vi "Thread@SubThreadSuspend__Parameter.vi"(1 "ParamterIn":string) -> (0 "ParamterOut":string)   [LabVIEW 2020]
panel:
  out "SubThread Name":string[](array[string])
  in  "ALL":bool
  in  "Thread Label":string(combo)
  in  "Confirm":bool
  # "Thread@SubThreadSuspend $SubName1(,$SubName2....)\nThread@SubThreadSuspend ALL\nThread@SubThreadSuspend ALL(,$SubName1,$SubName2....)"
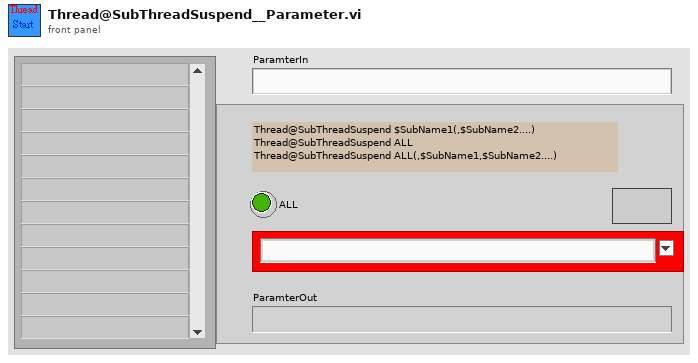
[diagram p1: front panel]
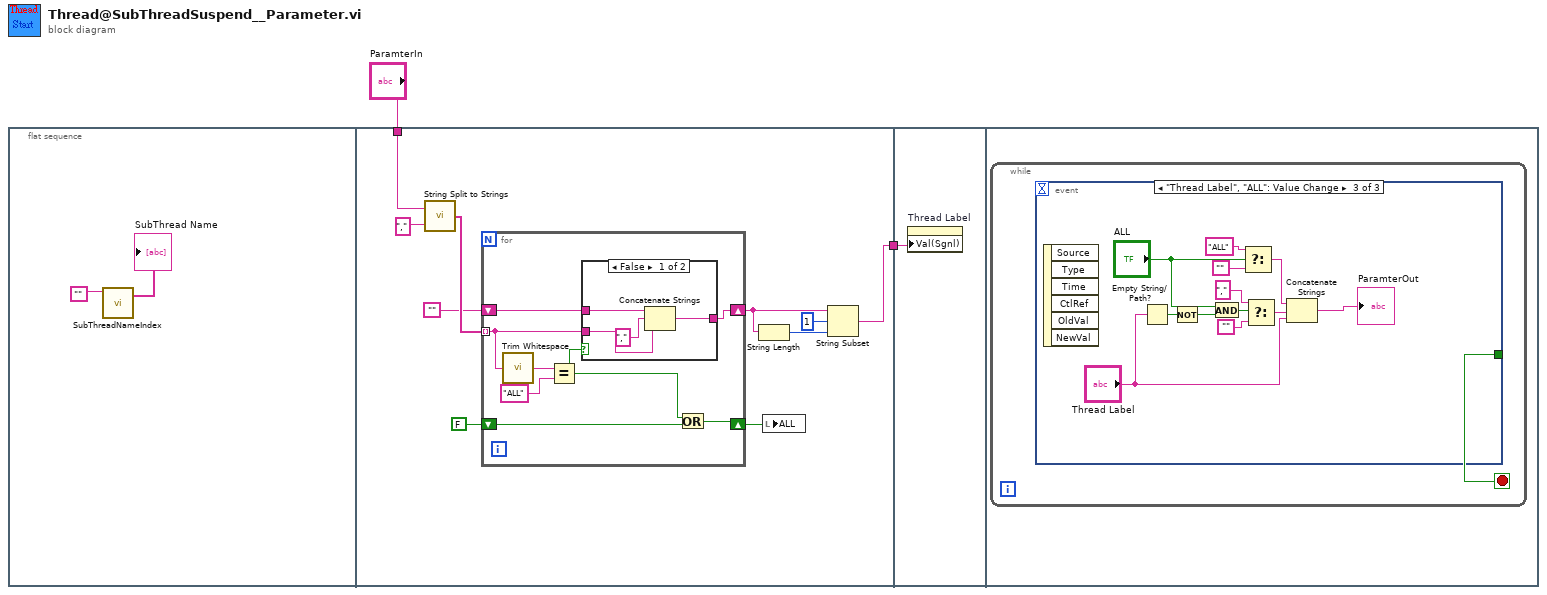
[diagram p0: block diagram]
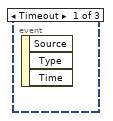
[diagram p3: hidden frame]
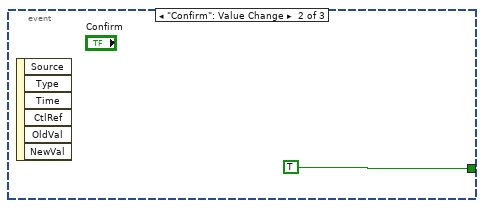
[diagram p4: hidden frame]
diagram:
  n1 = flat-sequence {
    tunnel: "ParamterIn" -> [w13]
    tunnel: [w7] -> w1
    tunnel: w1 -> [w28]
    frame #0 {
      n2 = call "SubThreadNameIndex.vi"("SubThreadName"="") -> ("SubThread Name"=→"SubThread Name":string[])  [unwired: 7 in, 3 out]
    }
    frame #1 {
      n3 = call "String Split to Strings.vi"("search string/char (-)"=",", "String"=w13) -> ("Array"=w12:string[])
      n4 = for {
        tunnel: w12 -> [w16] mode=indexing
        shift-right: [w15] -> w8
        shift-left: "" -> [w17]
        shift-right: [w20] -> w9
        shift-left: FALSE -> [w19]
        n5 = call <vilib>:"Trim Whitespace.vi"("string"=w16) -> ("trimmed string"=w22:string)  [unwired: 1 in]
        n6 = Equal?(x=w22, y="ALL") -> (x = y?=w18:bool)
        n7 = case shown="False" w18 {
          tunnel: w17 -> [w26 w27]
          tunnel: w16 -> [w23 _]
          tunnel: [w25 w27] -> w15
          frame False {
            n8 = Concatenate Strings(w26, ",", w23) -> (w25:string)
          }
          frame True {
          }
        }
        n9 = Or(x=w18, y=w19) -> (x .or. y?=w20:bool)
      }
      n10 = String Length(string=w8) -> (length=w6:i32)
      n11 = local write "ALL"(w9) -> ()
      n12 = String Subset(string=w8, offset (0)=1, length (rest)=w6) -> (substring=w7:string)
    }
    frame #2 {
      n13 = property on="Thread Label" class="CmbBox"("Val(Sgnl)"=w28) -> ()  [unwired: 2 in, 2 out]
    }
    frame #3 {
      n14 = while {
        stop <- w29 stop-if-true
        n15 = event shown="[2] \"Thread Label\", \"ALL\": Value Change" {
          selector: _ -> [_ _ _]
          dyn-events: _ -> [_ _ _]
          timeout: _ -> [_ _ _]
          tunnel: [_ TRUE _] -> w29
          event Timeout {
            n16 = event-data() -> ()  [unwired: 1 in, 3 out]
          }
          event "Confirm": Value Change {
            n17 = event-data() -> ()  [unwired: 1 in, 6 out]
          }
          event "Thread Label", "ALL": Value Change {
            n18 = event-data() -> ()  [unwired: 1 in, 6 out]
            n19 = Empty String/Path?(string/path="Thread Label") -> (empty?=w34:bool)
            n20 = Not(x=w34) -> (.not. x?=w33:bool)
            n21 = And(x="ALL", y=w33) -> (x .and. y?=w36:bool)
            n22 = Select(t="ALL", s="ALL", f="") -> (s? t:f=w40:string)
            n23 = Select(t=",", s=w36, f="") -> (s? t:f=w35:string)
            n24 = Concatenate Strings(w40, w35, "Thread Label") -> (→"ParamterOut":string)
          }
        }
      }
    }
  }
